vi "Display User Text Message.vi"(6 "Enable Lower Message (T: Enable)":bool=TRUE, 7 "Enable Upper Message (T: Enable)":bool=TRUE, 8 "error in (no error)":errorcluster, 9 "Lower Message (\"Message\")":string="\"Test running\"", 10 "Upper Message (\"Default\")":string="\"Batch A122\"", 11 "VISA resource name":refnum<visa-resource-name>) -> (0 "error out":errorcluster, 3 "VISA resource name out":refnum<visa-resource-name>)   [LabVIEW 2015, in "Keithley DMM6500 DAQ6500 Series.lvlib"]
doc: "Defines the text (both Top line and Bottom Line ) that is displayed on the front-panel USER swipe screen."
uses:
  <instrlib>/Keithley DMM6500 DAQ6500 Series/Keithley DMM6500 DAQ6500 Series.lvlib
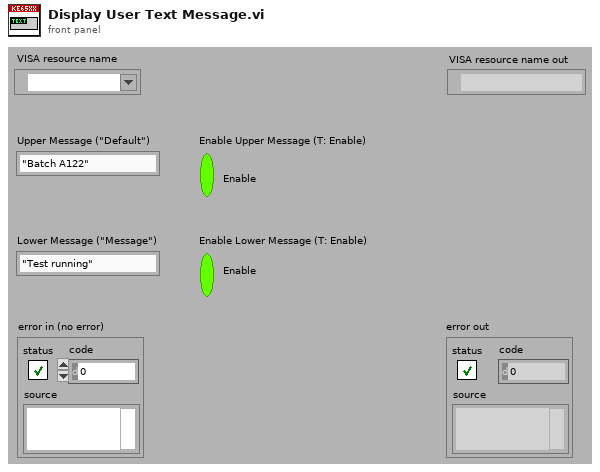
[diagram p1: front panel]
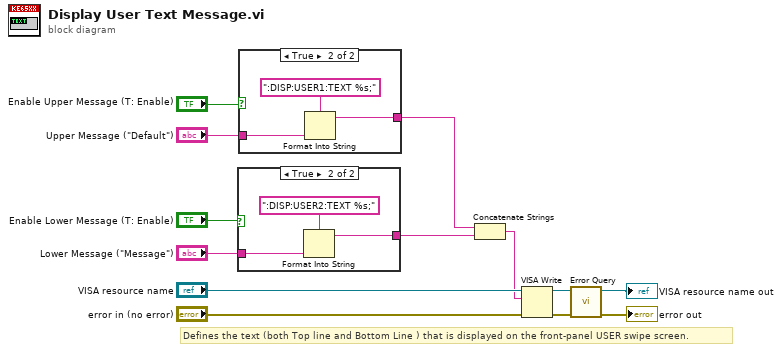
[diagram p0: block diagram]
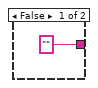
[diagram p2: hidden frame]
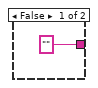
[diagram p3: hidden frame]
diagram:
  # "Defines the text (both Top line and Bottom Line ) that is displayed on the front-panel USER swipe screen."
  n1 = case shown="True" "Enable Lower Message (T: Enable)" {
    tunnel: ["" w17] -> w4
    tunnel: "Lower Message (\"Message\")" -> [_ w15]
    frame False {
    }
    frame True {
      n2 = Format Into String(format string=":DISP:USER2:TEXT %s;", w15) -> (resulting string=w17:string)  [unwired: 2 in, 1 out]
    }
  }
  n3 = case shown="True" "Enable Upper Message (T: Enable)" {
    tunnel: ["" w21] -> w1
    tunnel: "Upper Message (\"Default\")" -> [_ w19]
    frame False {
    }
    frame True {
      n4 = Format Into String(format string=":DISP:USER1:TEXT %s;", w19) -> (resulting string=w21:string)  [unwired: 2 in, 1 out]
    }
  }
  n5 = Concatenate Strings(w1, w4) -> (w5:string)
  n6 = VISA Write(VISA resource name="VISA resource name", write buffer=w5, error in (no error)="error in (no error)") -> (VISA resource name out=w11:refnum<visa-resource-name>, error out=w8:errorcluster)  [unwired: 1 out]
  n7 = call <instrlib>:"Error Query.vi"("error in (no error)"=w8, "VISA resource name"=w11) -> ("error out"=→"error out":errorcluster, "VISA resource name out"=→"VISA resource name out":refnum<visa-resource-name>)  [unwired: 6 in, 2 out]
